vi "SIM Calculate Machine Epsilon.vi"() -> (0 "min float":dbl, 1 "machine eps":dbl)   [LabVIEW 2020]
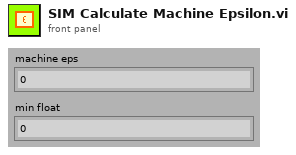
[diagram p1: front panel]
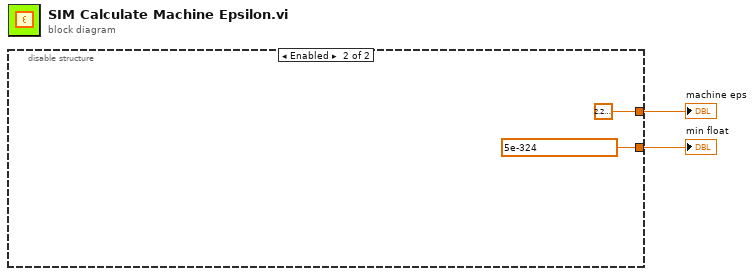
[diagram p0: block diagram]
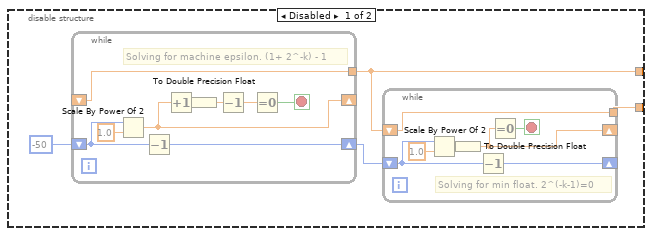
[diagram p2: hidden frame]
diagram:
  n1 = disable-structure shown="Enabled" {
    disable-tunnel: [w4 2.220446049250313e-16] -> w2
    disable-tunnel: [w3 5e-324 ("min float")] -> w1
    frame Disabled {
      n2 = while {
        shift-right: [w19] -> w6
        shift-left: -50 -> [w16]
        shift-right: [w15] -> _
        shift-left: _ -> [w18]
        tunnel: [w18] -> w4
        stop <- w22 stop-if-true
        # "Solving for machine epsilon. (1+ 2^-k) - 1"
        n3 = Scale By Power Of 2(n=w16, x=1.0) -> (x*2^n=w15:dbl)
        n4 = Decrement(x=w16) -> (x-1=w19:i32)
        n5 = Increment(x=w15) -> (x+1=w21:dbl)
        n6 = To Double Precision Float(number=w21) -> (double precision float=w14:dbl)
        n7 = Decrement(x=w14) -> (x-1=w20:dbl)
        n8 = Equal To 0?(x=w20) -> (x = 0?=w22:bool)
      }
      n9 = while {
        shift-right: [w10] -> _
        shift-left: w6 -> [w11]
        shift-right: [w7] -> _
        shift-left: w4 -> [w13]
        tunnel: [w13] -> w3
        stop <- w9 stop-if-true
        # "Solving for min float. 2^(-k-1)=0"
        n10 = Scale By Power Of 2(n=w11, x=1.0) -> (x*2^n=w8:dbl)
        n11 = To Double Precision Float(number=w8) -> (double precision float=w7:dbl)
        n12 = Decrement(x=w11) -> (x-1=w10:i32)
        n13 = Equal To 0?(x=w7) -> (x = 0?=w9:bool)
      }
    }
    frame Enabled {
    }
  }
  "machine eps" <- w2
  "min float" <- w1
